vi "Check Slave ID.vi"(8 "error in (no error)":errorcluster, 9 "Slave ID in":u16, 11 "Item Ref in":T1 format="%.0x") -> (0 "error out":errorcluster, 1 "Slave ID out":u16, 2 "Available?":bool, 3 "Item Ref out":T1 format="%.0x")   [LabVIEW 2019, in "Scan Engine Custom Device.lvlib"]
uses:
  Scan Engine Custom Device.lvlib
  <vilib>/NI VeriStand/Custom Device API/Custom Device Item Ref.ctl
  <vilib>/NI VeriStand/Custom Device API/Custom Device API.lvlib
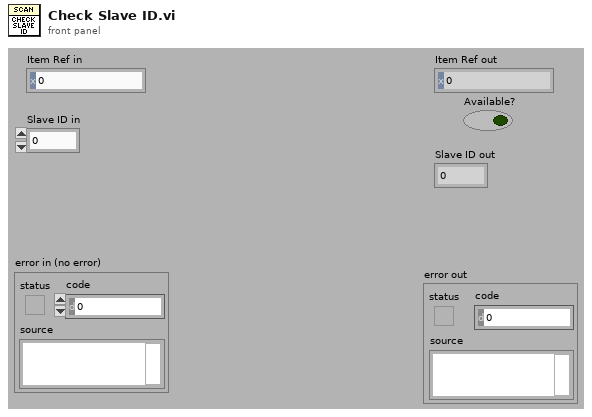
[diagram p1: front panel]
types:
  T1 = typedef "Custom Device API.lvlib/Custom Device Item Ref.ctl" = u64
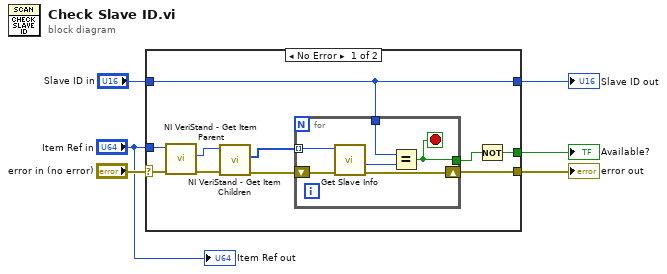
[diagram p0: block diagram]
diagram:
  n1 = case shown="No Error" "error in (no error)" {
    selector: "error in (no error)" -> [w9 w24]
    tunnel: [w13 w24] -> w5
    tunnel: "Item Ref in" -> [w10 _]
    tunnel: "Slave ID in" -> [w12 w23]
    tunnel: [w12 w23] -> w3
    tunnel: [w11 _] -> w2
    frame No Error {
      n2 = call <vilib>:"NI VeriStand - Get Item Parent.vi"("error in (no error)"=w9, "Item Ref in"=w10) -> ("error out"=w8:errorcluster, "Parent Ref"=w7:T1)  [unwired: 6 in, 2 out]
      n3 = call <vilib>:"NI VeriStand - Get Item Children.vi"("error in (no error)"=w8, "Item Ref in"=w7) -> ("error out"=w16:errorcluster, "Child Refs"=w15:T1[])  [unwired: 6 in, 2 out]
      n4 = for {
        tunnel: w15 -> [w19] mode=indexing
        shift-right: [w18] -> w13
        shift-left: w16 -> [w20]
        tunnel: w12 -> [w22]
        tunnel: [w21] -> w14
        stop <- w21 stop-if-true
        n5 = call "Get Slave Info.vi"("error in (no error)"=w20, "Item Ref in"=w19) -> ("error out"=w18:errorcluster, "Slave #"=w17:u16)  [unwired: 5 in, 3 out]
        n6 = Equal?(x=w22, y=w17) -> (x = y?=w21:bool)
      }
      n7 = Not(x=w14) -> (.not. x?=w11:bool)
    }
    frame Error {
    }
  }
  "error out" <- w5
  "Available?" <- w2
  "Slave ID out" <- w3
  "Item Ref out" <- "Item Ref in"
